vi "GUI Notifier Wait for Message.vi"(7 "last state":string, 8 "error in (no error)":errorcluster, 9 "cases to ignore":string[](array[string]), 10 "acquisition states":string[](array[string]), 11 "gui notifier":refnum<notifier>) -> (0 "error out":errorcluster, 3 "gui msg":string)   [LabVIEW 2020]
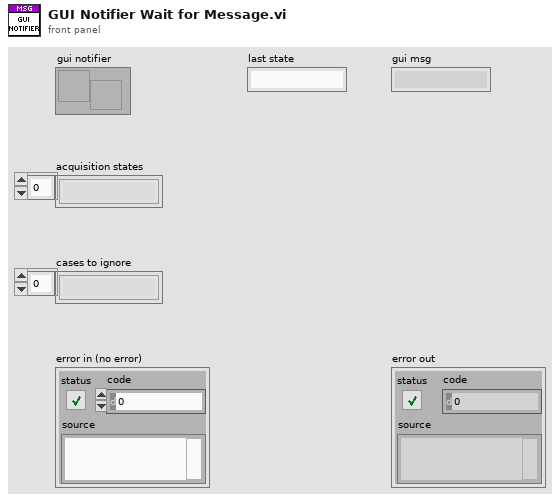
[diagram p1: front panel]
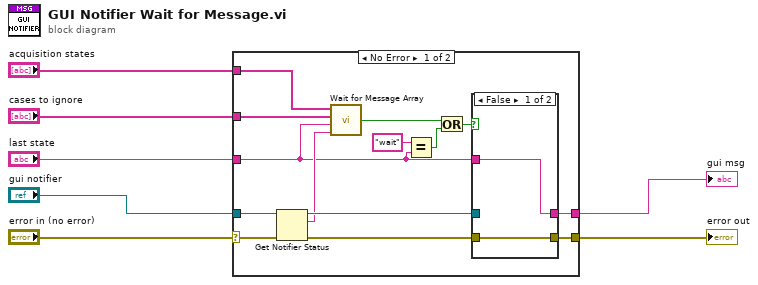
[diagram p0: block diagram]
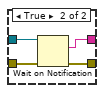
[diagram p2: hidden frame]
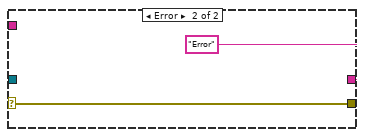
[diagram p3: hidden frame]
diagram:
  n1 = case shown="No Error" "error in (no error)" {
    selector: "error in (no error)" -> [w19 w29]
    tunnel: "gui notifier" -> [w17 _]
    tunnel: [w21 w29] -> w2
    tunnel: [w20 "Error" ("gui msg")] -> w7
    tunnel: "last state" -> [w9 _]
    tunnel: "cases to ignore" -> [w14 _]
    tunnel: "acquisition states" -> [w13 _]
    frame No Error {
      n2 = Get Notifier Status(notifier=w17, error in (no error)=w19) -> (notifier out=w16:refnum<notifier>, current notification=w15:string, error out=w18:errorcluster)  [unwired: 2 out]
      n3 = call "Wait for Message Array.vi"("gui notification"=w15, "last state"=w9, "cases to ignore"=w14, "acquisition state array"=w13) -> ("wait for message?"=w12:bool)
      n4 = Equal?(x="wait", y=w9) -> (x = y?=w10:bool)
      n5 = Or(x=w12, y=w10) -> (x .or. y?=w11:bool)
      n6 = case shown="False" w11 {
        tunnel: w16 -> [_ w27]
        tunnel: [w23 w26] -> w21
        tunnel: w18 -> [w23 w25]
        tunnel: [w22 w24] -> w20
        tunnel: w9 -> [w22 _]
        frame False {
        }
        frame True {
          n7 = Wait on Notification(notifier=w27, error in (no error)=w25) -> (notification=w24:string, error out=w26:errorcluster)  [unwired: 2 in, 2 out]
        }
      }
    }
    frame Error {
    }
  }
  "gui msg" <- w7
  "error out" <- w2
